vi "conpane_test.vi"(9 "Numeric 3":dbl, 11 "Numeric":dbl) -> (2 "Numeric 2":dbl)   [LabVIEW 2012]
uses:
  Term Types.ctl
  Term Type.ctl
panel:
  in  "conpane_test.vi":T1
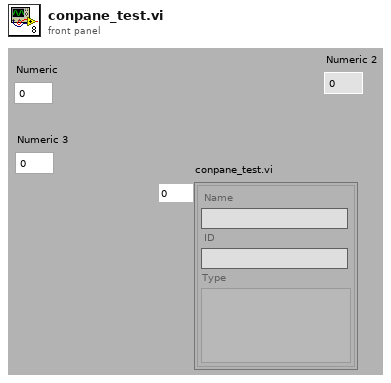
[diagram p1: front panel]
types:
  T1 = typedef "Term Types.ctl" = T2[]
  T2 = typedef "Term Type.ctl" = cluster{"Name":string, "ID":string, "Type":variant}
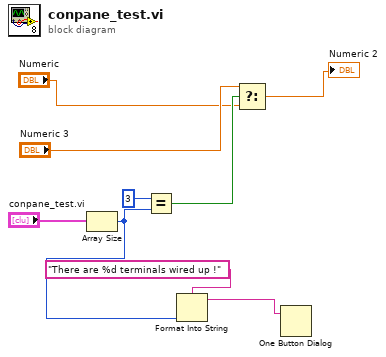
[diagram p0: block diagram]
diagram:
  n1 = Array Size(array="conpane_test.vi") -> (size(s)=w2:i32)
  n2 = Equal?(x=3, y=w2) -> (x = y?=w7:bool)
  n3 = Format Into String(format string="There are %d terminals wired up !", w2) -> (resulting string=w1:string)  [unwired: 2 in, 1 out]
  n4 = Select(t="Numeric 3", s=w7, f="Numeric") -> (s? t:f=→"Numeric 2":dbl)
  n5 = One Button Dialog(message=w1) -> ()  [unwired: 2 out]
